vi "Set DDG Gate Time.vi"(8 "error in (no error)":errorcluster, 10 "uiWidth":cluster{}, 11 "uiDelay":cluster{}) -> (0 "error out":errorcluster, 3 "function return":u32)   [LabVIEW 2014, in "atmcd32d.lvlib"]
doc: "unsigned int WINAPI SetDDGGateTime(at_u64 uiDelay, at_u64 uiWidth);"
uses:
  atmcd32d.lvlib
  atmcd32d.dll
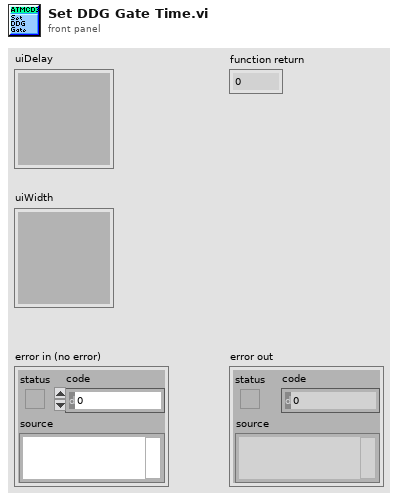
[diagram p1: front panel]
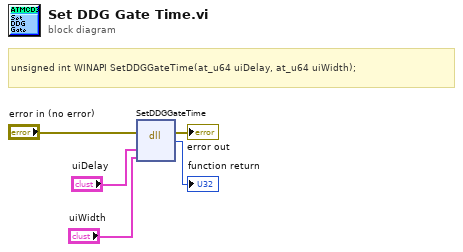
[diagram p0: block diagram]
diagram:
  # "unsigned int WINAPI SetDDGGateTime(at_u64 uiDelay, at_u64 uiWidth);"
  n1 = dll-call lib="C:/Users/Bakir/Documents/Lambda2-Testing/lib/Andorlib/atmcd32d.*" fn="SetDDGGateTime"(error in="error in (no error)", "uiDelay"="uiDelay", "uiWidth"="uiWidth") -> (error out=→"error out":errorcluster, →"function return":u32)  [unwired: 4 in, 1 out]
